vi "ListAllBuildSpecs.vi"(8 "error in (no error)":errorcluster, 11 "CommandLine":string[](array[string])) -> (0 "error out":errorcluster, 2 "test details":string)   [LabVIEW 2019]
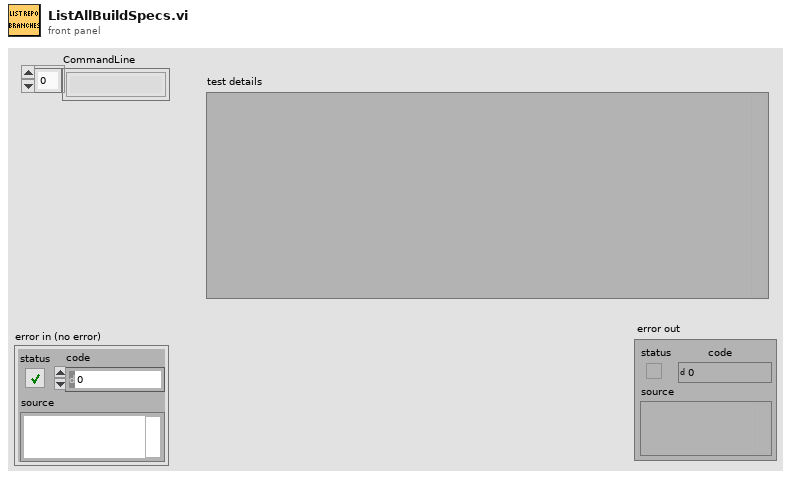
[diagram p1: front panel]
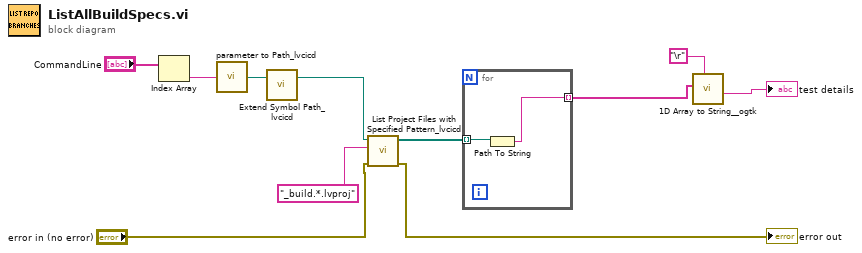
[diagram p0: block diagram]
diagram:
  n1 = Index Array(array="CommandLine") -> (element=w8:string)  [unwired: 1 in]
  n2 = call "parameter to Path_lvcicd.vi"("String"=w8) -> ("Path"=w11:path)
  n3 = call "Extend Symbol Path_lvcicd.vi"("Symbol Path"=w11) -> ("Resolved Path"=w6:path)  [unwired: 2 in]
  n4 = call "List Project Files with Specified Pattern_lvcicd.vi"("error in (no error)"="error in (no error)", "pattern"="_build.*.lvproj", "Path"=w6) -> ("error out"=→"error out":errorcluster, "All Files in Dir"=w3:path[])  [unwired: 6 in, 1 out]
  n5 = for {
    tunnel: w3 -> [w13] mode=indexing
    tunnel: [w12] -> w2 mode=indexing
    n6 = Path To String(path=w13) -> (string=w12:string)
  }
  n7 = call <userlib>:"1D Array to String__ogtk.vi"("delimiter (Tab)"="\r", "Array of Strings"=w2) -> ("delimited string"=→"test details":string)  [unwired: 9 in]
